vi "APC_9049_HRL_IMEP.vi"(0 "Volume cluster":T1, 1 "Pressure":dbl[](array[numeric])) -> (2 "IMPEn":dbl, 3 "IMEPg":dbl, 4 "Pmax":dbl, 5 "PMEP":dbl)   [LabVIEW 2020]
uses:
  controls/APC_volume.ctl
  <vilib>/Analysis/8numeric.llb/1D Numeric Integration.vi
  <vilib>/Analysis/NI_AALPro.lvlib
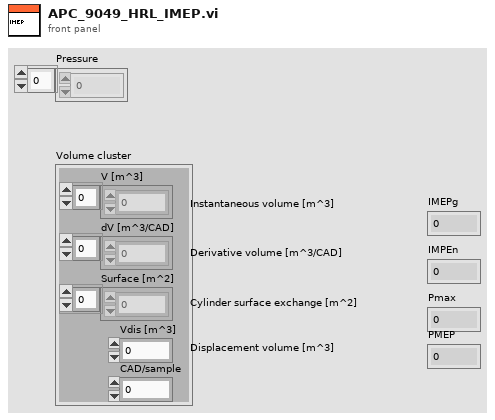
[diagram p1: front panel]
types:
  T1 = typedef "APC_volume.ctl" = cluster{"V [m^3]":dbl[], "dV [m^3/CAD]":dbl[], "Vdis [m^3]":dbl, "Surface [m^2]":dbl[], "CAD/sample":dbl}
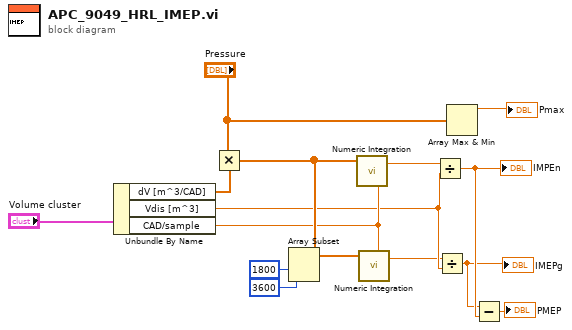
[diagram p0: block diagram]
diagram:
  n1 = Unbundle By Name("Volume cluster") -> ("dV [m^3/CAD]"=w6:dbl[], "Vdis [m^3]"=w9:dbl, "CAD/sample"=w10:dbl)
  n2 = Multiply(x="Pressure", y=w6) -> (x*y=w11:dbl[])
  n3 = Array Subset(array=w11, index=1800, length=3600) -> (w14:dbl[])
  n4 = call-poly <vilib>:"Numeric Integration.vi"("dt"=w10, "Input Array"=w11) -> ("result"=w7:dbl)  [unwired: 1 in, 1 out]
  n5 = call-poly <vilib>:"Numeric Integration.vi"("dt"=w10, "Input Array"=w14) -> ("result"=w8:dbl)  [unwired: 1 in, 1 out]
  n6 = Divide(x=w7, y=w9) -> (x/y=w2:dbl)
  "IMPEn" <- w2
  n7 = Divide(x=w8, y=w9) -> (x/y=w1:dbl)
  "IMEPg" <- w1
  n8 = Array Max & Min(array="Pressure") -> (max value=→"Pmax":dbl)  [unwired: 3 out]
  n9 = Subtract(x=w1, y=w2) -> (x-y=→"PMEP":dbl)
